vi "Load PPL Versions.vi"(8 "error in":errorcluster, 11 "Module Plugin Directory":path=path "/home/lvuser/natinst/bin") -> (0 "error out":errorcluster, 1 "Plugin Objects":refnum<class "PowerModuleInterface.lvclass">[](array[class]), 2 "Plugin Names":string[](array[string]), 3 "Plugin Versions":string[](array[string]))   [LabVIEW 2023]
uses:
  <vilib>/Utility/LVLibp/NI_PackedLibraryUtility.lvlib
  builds/PowerModuleInterface/home/lvuser/natinst/bin/PowerModuleInterface.lvlibp/Classes/PowerModule_interface/PowerModuleInterface.lvclass
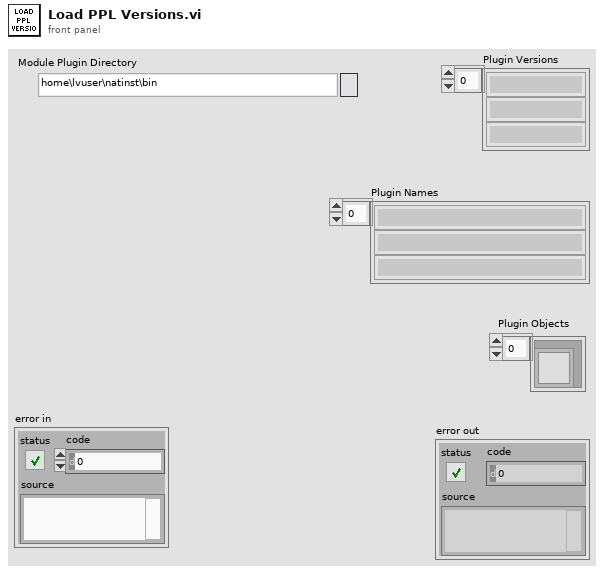
[diagram p1: front panel]
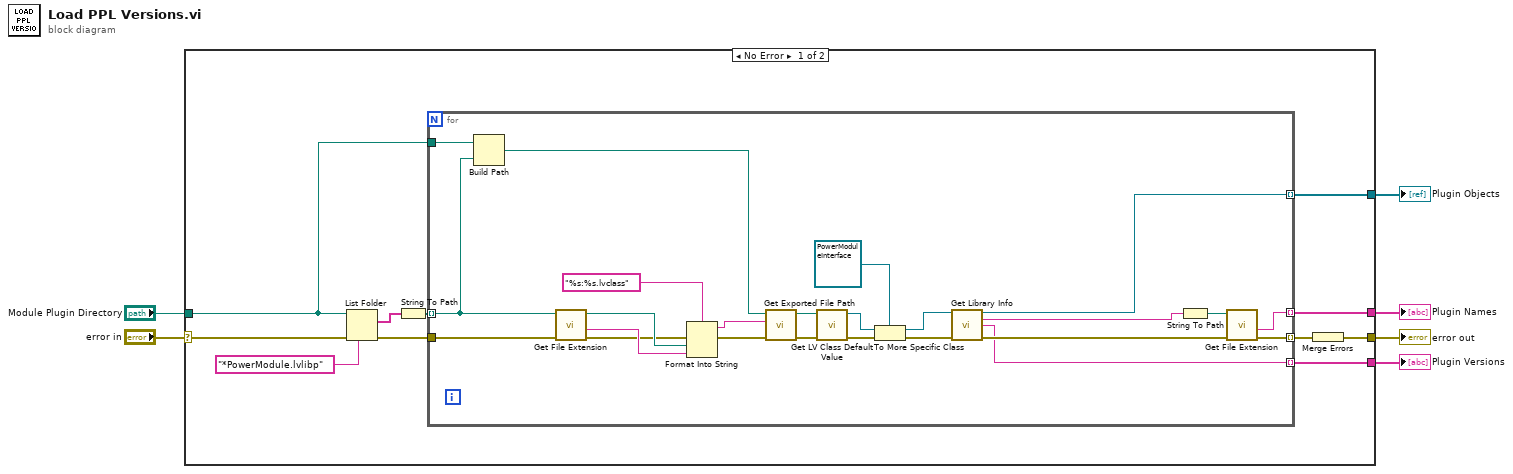
[diagram p0: block diagram]
diagram:
  n1 = case shown="No Error" "error in" {
    selector: "error in" -> [w9 w42]
    tunnel: [w12 w42] -> w6
    tunnel: [w11 _] -> w5
    tunnel: [w10 _] -> w4
    tunnel: "Module Plugin Directory" -> [w7 _]
    tunnel: [w8 _] -> w1
    frame No Error {
      n2 = List Folder(path=w7, pattern="*PowerModule.lvlibp", error in=w9) -> (filenames=w15:string[], error out=w16:errorcluster)  [unwired: 1 in, 2 out]
      n3 = String To Path(string=w15) -> (path=w14:path[])
      n4 = for {
        tunnel: w16 -> [w41]
        tunnel: w14 -> [w36] mode=indexing
        tunnel: [w38] -> w13 mode=indexing
        tunnel: [w18] -> w11 mode=indexing
        tunnel: [w40] -> w10 mode=indexing
        tunnel: [w20] -> w8 mode=indexing
        tunnel: w7 -> [w37]
        n5 = Build Path(base path=w37, name or relative path=w36) -> (appended path=w29:path)
        n6 = call <vilib>:"Get File Extension.vi"("error in (no error)"=w41, "file"=w36) -> ("error out"=w32:errorcluster, "filename without extension"=w33:string, "dup file"=w34:path)  [unwired: 5 in, 2 out]
        n7 = Format Into String(format string="%s:%s.lvclass", error in=w32, w34, w33) -> (resulting string=w30:string, error out=w31:errorcluster)  [unwired: 1 in]
        n8 = call <vilib>:"Get Exported File Path.vi"("error in (no error)"=w31, "qualified name"=w30, "packed library path"=w29) -> ("error out"=w28:errorcluster, "path"=w27:path)  [unwired: 7 in]
        n9 = call <vilib>:"Get LV Class Default Value.vi"("error in (no error)"=w28, "class path"=w27) -> ("error out"=w26:errorcluster, "object"=w25:refnum<class>)  [unwired: 8 in]
        n10 = To More Specific Class(target class=refnum<class "PowerModuleInterface.lvclass"> refnum ("object in"), reference=w25, error in=w26) -> (specific class reference=w22:refnum<class "PowerModuleInterface.lvclass">, error out=w23:errorcluster)
        n11 = call-dynamic "Get Library Info.vi"("object in"=w22, "Error In"=w23) -> ("object out"=w20:refnum<class "PowerModuleInterface.lvclass">, "PPL Filename"=w19:string, "Build Version"=w18:string, "Error Out"=w21:errorcluster)  [unwired: 10 in]
        n12 = String To Path(string=w19) -> (path=w39:path)
        n13 = call <vilib>:"Get File Extension.vi"("error in (no error)"=w21, "file"=w39) -> ("error out"=w38:errorcluster, "filename without extension"=w40:string)  [unwired: 5 in, 3 out]
      }
      n14 = Merge Errors(w13) -> (w12:errorcluster)
    }
    frame Error {
    }
  }
  "error out" <- w6
  "Plugin Versions" <- w5
  "Plugin Names" <- w4
  "Plugin Objects" <- w1
